vi "signal_level.vi"(5 "data U16":u16[](array[numeric]), 9 "signal?":bool=TRUE) -> (6 "level":T1={"Slide 5"={1482, 2181}, "max OL 10"=FALSE, "max OL 9"=FALSE, "Slide 4"={1477, 2189}, "max OL 8"=FALSE, "max OL 7"=FALSE} {"Slide 4" scale=0.0..4096.0; "Slide 5" scale=0.0..4096.0})   [LabVIEW 2017, in "ZBOX_IS.lvlib"]
uses:
  ZBOX_IS.lvlib
panel:
  out "Array":u16[](array[numeric])
  out "max OL 7":bool
  out "max OL 8":bool
  out "Slide 4":cluster{u16, u16}(slide)={1477, 2189} scale=0.0..4096.0
  out "max OL 9":bool
  out "max OL 10":bool
  out "Slide 5":cluster{u16, u16}(slide)={1482, 2181} scale=0.0..4096.0
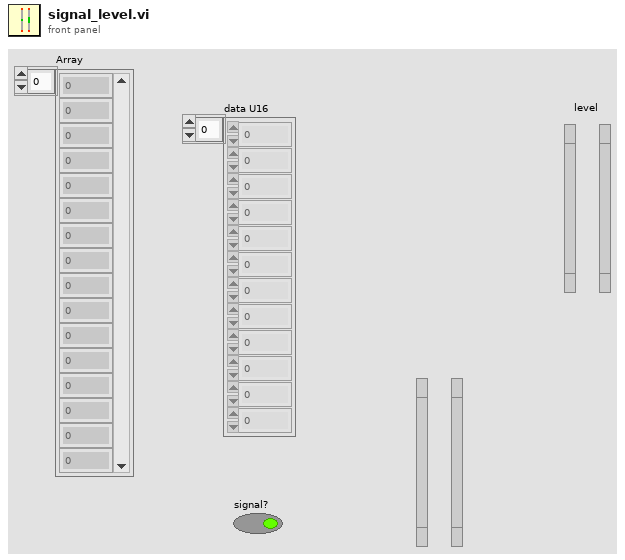
[diagram p1: front panel]
types:
  T1 = cluster{"Slide 5":cluster{u16, u16}, "max OL 10":bool, "max OL 9":bool, "Slide 4":cluster{u16, u16}, "max OL 8":bool, "max OL 7":bool}
  T2 = cluster{cluster{u16, u16}, bool, bool, cluster{u16, u16}, bool, bool}
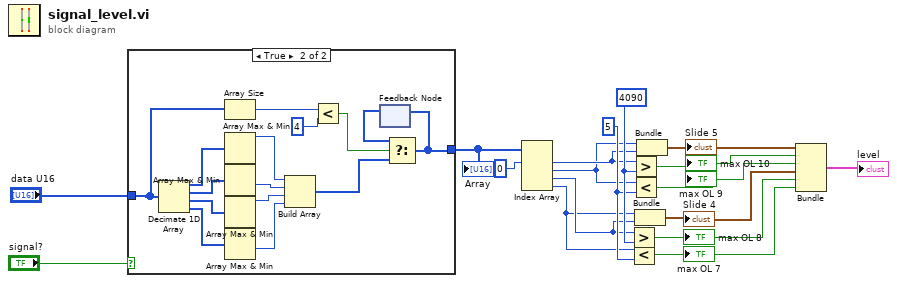
[diagram p0: block diagram]
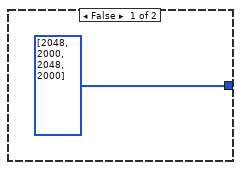
[diagram p2: hidden frame]
diagram:
  w16 = u16 5 ("y")
  w17 = u16 4090 ("y")
  n1 = case shown="True" "signal?" {
    tunnel: "data U16" -> [_ w19]
    tunnel: [u16[] [2048, 2000, 2048, 2000] w20] -> w1
    frame False {
    }
    frame True {
      n2 = Decimate 1D Array(w19) -> (w26:u16[], w27:u16[], w28:u16[], w29:u16[])
      n3 = Array Size(array=w19) -> (size(s)=w23:i32)
      n4 = Array Max & Min(array=w26) -> (max value=w30:u16)  [unwired: 3 out]
      n5 = Array Max & Min(array=w27) -> (min value=w31:u16)  [unwired: 3 out]
      n6 = Array Max & Min(array=w28) -> (max value=w32:u16)  [unwired: 3 out]
      n7 = Array Max & Min(array=w29) -> (min value=w33:u16)  [unwired: 3 out]
      n8 = Build Array(w30, w31, w32, w33) -> (w25:u16[])
      n9 = Less?(x=w23, y=4) -> (x < y?=w21:bool)
      n10 = feedback #1() -> (w24:u16[])  [unwired: 1 in]
      n11 = Select(t=w24, s=w21, f=w25) -> (s? t:f=w20:u16[])
      n12 = feedback-in #1(w20) -> ()
    }
  }
  "Array" <- w1
  n13 = Index Array(array=w1, index #1=0 ("index")) -> (element #1=w13:u16, element #2=w12:u16, element #3=w15:u16, element #4=w14:u16)  [unwired: 3 in]
  n14 = Greater?(x=w15, y=w17) -> (0:w7:bool)
  "max OL 8" <- w7
  n15 = Less?(x=w14, y=w16) -> (x < y?=w6:bool)
  "max OL 7" <- w6
  n16 = Greater?(x=w13, y=w17) -> (0:w10:bool)
  "max OL 10" <- w10
  n17 = Less?(x=w12, y=w16) -> (x < y?=w9:bool)
  "max OL 9" <- w9
  n18 = Bundle(w14, w15) -> (w8:cluster{u16, u16})  [unwired: 1 out]
  "Slide 4" <- w8
  n19 = Bundle(w12, w13) -> (w11:cluster{u16, u16})  [unwired: 1 out]
  "Slide 5" <- w11
  n20 = Bundle(w11, w10, w9, w8, w7, w6) -> (→"level":T2)  [unwired: 1 in]
